vi "Begin-End.vi"(8 "Error In":errorcluster) -> (0 "Error Out":errorcluster)   [LabVIEW 2018, in "Tests.lvlib" / "Reader.lvlib"]
uses:
  Reader.lvlib
  src/Toolkit/Public/Reader/Private/Begin by Value.vi
  src/Toolkit/Public/Reader/Private/End by Value.vi
  <vilib>/addons/_JKI Toolkits/Caraya/classes/Test/Test.lvclass
  src/Toolkit/Public/Reader/Reader.lvclass
  <vilib>/addons/_JKI Toolkits/Caraya/classes/Assert/Assert.lvclass
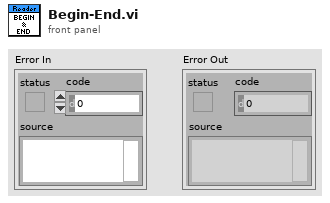
[diagram p1: front panel]
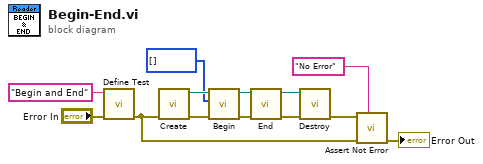
[diagram p0: block diagram]
diagram:
  n1 = call <vilib>:"Define Test.vi"("error in (no error)"="Error In", "Label (VI Title)"="Begin and End") -> ("error out"=w3:errorcluster)  [unwired: 9 in]
  n2 = call "Create.vi"("Error In"=w3) -> ("Error Out"=w11:errorcluster, "Reader"=w10:refnum<class "Reader.lvclass">)  [unwired: 9 in]
  n3 = call-poly "Begin.vi"("Error In"=w11, "Msgpack Data"=u8[] [], "Reader In"=w10) -> ("Error Out"=w8:errorcluster, "Reader Out"=w9:refnum<class "Reader.lvclass">)  [unwired: 7 in]
  n4 = call-poly "End.vi"("Error In"=w8, "Reader In"=w9) -> ("Error Out"=w6:errorcluster, "Reader Out"=w7:refnum<class "Reader.lvclass">)  [unwired: 8 in]
  n5 = call "Destroy.vi"("Error In"=w6, "Reader"=w7) -> ("Error Out"=w5:errorcluster)  [unwired: 9 in]
  n6 = call <vilib>:"Assert Not Error.vi"("Label"="No Error", "error in (no error)"=w3, "Not Error?"=w5) -> ("error out"=→"Error Out":errorcluster)  [unwired: 8 in]
